vi "getCamRamMaxImages.vi"(0 "Camera in":refnum<class "Camera.lvclass">, 11 "error in (no error)":errorcluster) -> (4 "Camera out":refnum<class "Camera.lvclass">, 6 "max_images":u32, 15 "error out":errorcluster)   [LabVIEW 2019, in "Camera.lvclass"]
doc: "Determines the maximum number of images that can be stored in the current camera RAM segment. For cameras with internal memory only. Returns an error if camera does not have internal memory."
uses:
  Camera.lvclass
  Camera.lvclass/Camera.ctl
  pco.sdk/ImageInformation/ImageInformation.lvlib
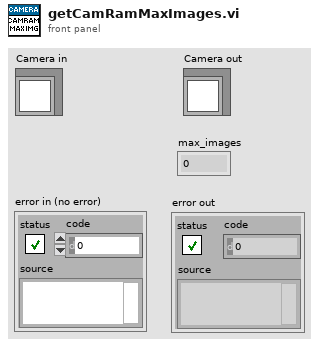
[diagram p1: front panel]
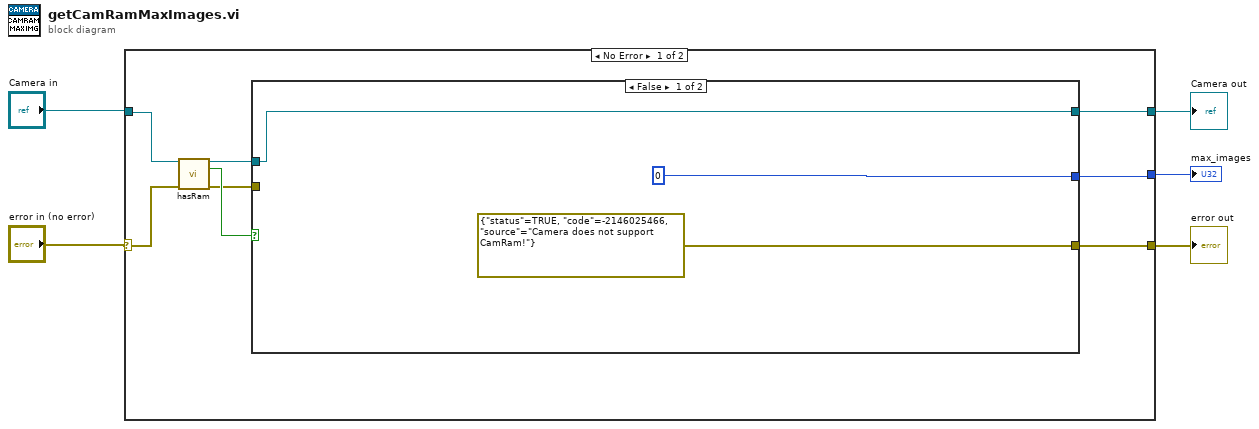
[diagram p0: block diagram]
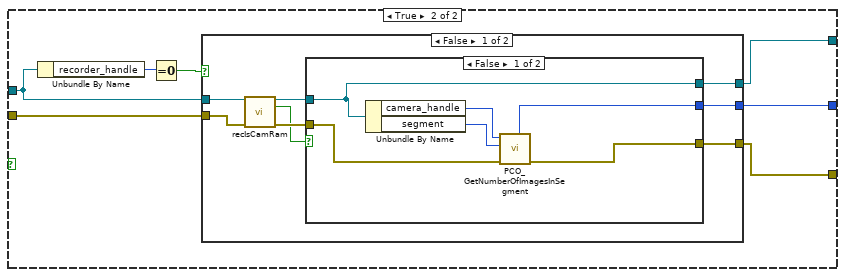
[diagram p2: hidden frame]
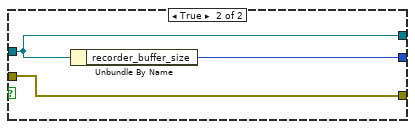
[diagram p3: hidden frame]
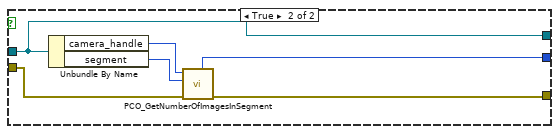
[diagram p4: hidden frame]
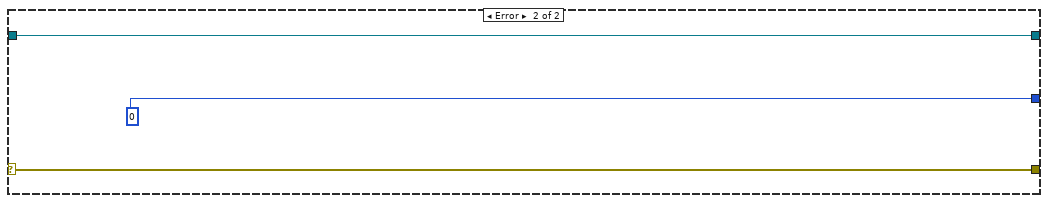
[diagram p5: hidden frame]
diagram:
  n1 = case shown="No Error" "error in (no error)" {
    selector: "error in (no error)" -> [w10 w49]
    tunnel: [w6 w49] -> w3
    tunnel: [w8 w48] -> w4
    tunnel: "Camera in" -> [w9 w48]
    tunnel: [w7 u32 0 ("dwErr")] -> w1
    frame No Error {
      n2 = call-dynamic "hasRam.vi"("Camera in"=w9, "error in (no error)"=w10) -> ("Camera out"=w11:refnum<class "Camera.lvclass">, "hasRam"=w13:bool, "error out"=w12:errorcluster)  [unwired: 11 in]
      n3 = case shown="False" w13 {
        tunnel: w11 -> [w14 w21]
        tunnel: [errorcluster {"status"=TRUE, "code"=-2146025466, "source"="Camera does not support CamRam!"} ("error constant") w19] -> w6
        tunnel: w12 -> [_ w20]
        tunnel: [w14 w18] -> w8
        tunnel: [u32 0 ("dwMaxImageCnt") w17] -> w7
        frame False {
        }
        frame True {
          n4 = Unbundle By Name(w21) -> ("recorder_handle"=w23:u64)
          n5 = Equal To 0?(x=w23) -> (x = 0?=w22:bool)
          n6 = case shown="False" w22 {
            tunnel: w21 -> [w31 w42]
            tunnel: w20 -> [w30 w46]
            tunnel: [w24 w43] -> w19
            tunnel: [w26 w42] -> w18
            tunnel: [w25 w41] -> w17
            frame False {
              n7 = call-dynamic "recIsCamRam.vi"("Camera in"=w31, "error in (no error)"=w30) -> ("Camera out"=w28:refnum<class "Camera.lvclass">, "isCamram"=w27:bool, "error out"=w29:errorcluster)  [unwired: 11 in]
              n8 = case shown="False" w27 {
                tunnel: w29 -> [w35 w38]
                tunnel: w28 -> [w33 w40]
                tunnel: [w33 w40] -> w26
                tunnel: [w34 w39] -> w25
                tunnel: [w32 w38] -> w24
                frame False {
                  n9 = Unbundle By Name(w33) -> ("camera_handle"=w37:u64, "segment"=w36:u16)
                  n10 = call "PCO_GetNumberOfImagesInSegment.vi"("error in (no error)"=w35, "wSegment"=w36, "ph"=w37) -> ("error out"=w32:errorcluster, "dwMaxImageCnt"=w34:u32)  [unwired: 4 in, 3 out]
                }
                frame True {
                  n11 = Unbundle By Name(w40) -> ("recorder_buffer_size"=w39:u32)
                }
              }
            }
            frame True {
              n12 = Unbundle By Name(w42) -> ("camera_handle"=w45:u64, "segment"=w44:u16)
              n13 = call "PCO_GetNumberOfImagesInSegment.vi"("error in (no error)"=w46, "wSegment"=w44, "ph"=w45) -> ("error out"=w43:errorcluster, "dwMaxImageCnt"=w41:u32)  [unwired: 4 in, 3 out]
            }
          }
        }
      }
    }
    frame Error {
    }
  }
  "error out" <- w3
  "Camera out" <- w4
  "max_images" <- w1
